vi "Close.vi"(8 "error in (no error)":errorcluster, 11 "LoggingHandle in":refnum<class "LoggingHandle.lvclass">) -> (0 "error out":errorcluster)   [LabVIEW 2024, in "LoggingHandle.lvclass"]
uses:
  LoggingHandle.lvclass
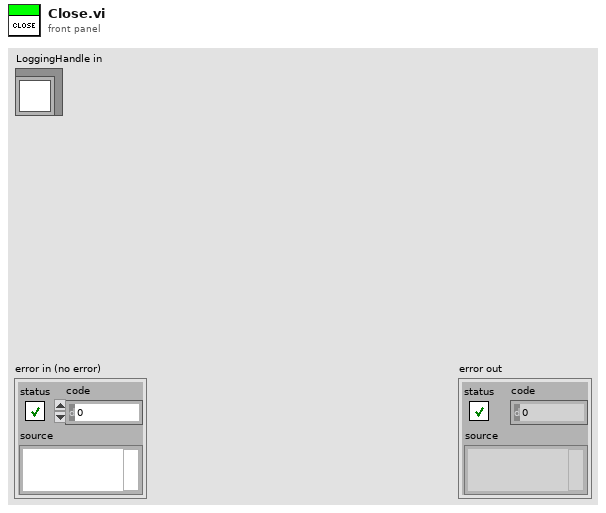
[diagram p1: front panel]
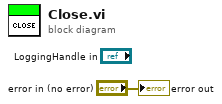
[diagram p0: block diagram]
diagram:
  "error out" <- "error in (no error)"
